vi "Clear Action Core.vi"(8 "error in (no error)":errorcluster, 11 "NI DAQmx AI Voltage in":refnum<class "NI DAQmx AI Voltage.lvclass">) -> (0 "error out":errorcluster, 3 "NI DAQmx AI Voltage out":refnum<class "NI DAQmx AI Voltage.lvclass">)   [LabVIEW 2020, in "NI DAQmx AI Voltage.lvlib" / "NI DAQmx AI Voltage.lvclass"]
uses:
  NI DAQmx AI Voltage.lvclass
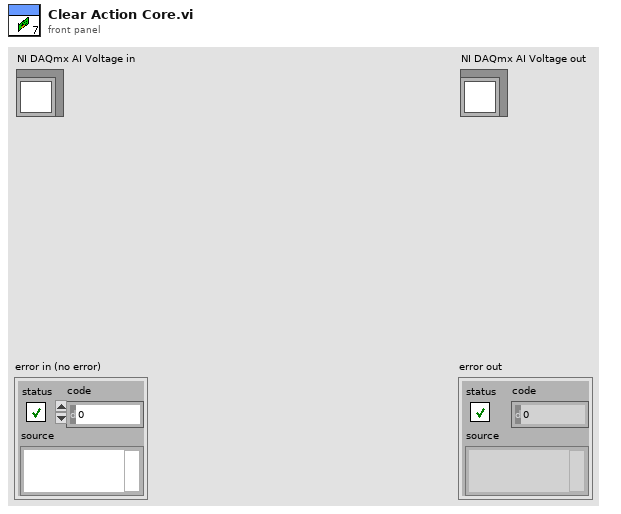
[diagram p1: front panel]
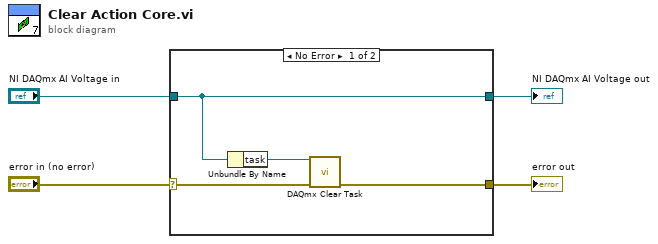
[diagram p0: block diagram]
diagram:
  n1 = case shown="No Error" "error in (no error)" {
    selector: "error in (no error)" -> [w8 w10]
    tunnel: "NI DAQmx AI Voltage in" -> [w6 w9]
    tunnel: [w5 w10] -> w1
    tunnel: [w6 w9] -> w3
    frame No Error {
      n2 = Unbundle By Name(w6) -> ("task"=w7:refnum<k21>)
      n3 = call <vilib>:"DAQmx Clear Task.vi"("task in"=w7, "error in"=w8) -> ("error out"=w5:errorcluster)  [unwired: 13 in]
    }
    frame Error {
    }
  }
  "error out" <- w1
  "NI DAQmx AI Voltage out" <- w3
